vi "Take single measurement.vi"() -> ()   [LabVIEW 2017, in "GP22_TDC_Arduinoed.lvlib"]
uses:
  GP22_TDC_Arduinoed.lvlib
panel:
  out "error out":errorcluster
  out "Calibration / s":dbl format="%^#_6g"
  out "output / s":dbl format="%^#_6g"
  out "Self-Test Result Message":string
  in  "VISA resource name":refnum<visa-resource-name>
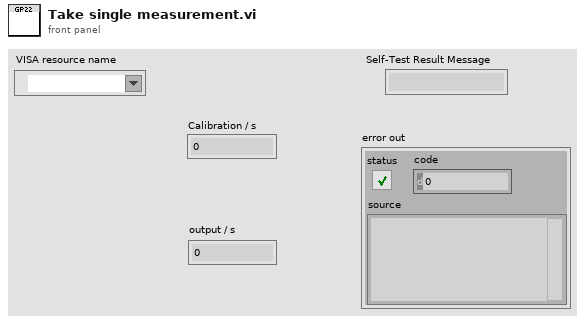
[diagram p1: front panel]
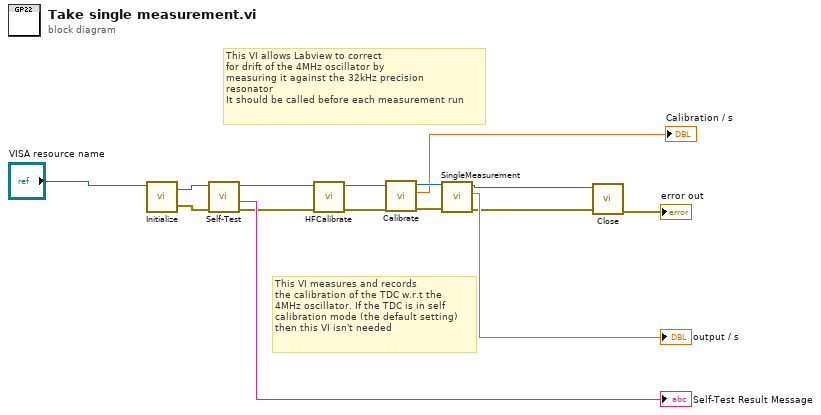
[diagram p0: block diagram]
diagram:
  # "This VI measures and records\nthe calibration of the TDC w.r.t the \n4MHz oscillator. If the TDC is in self \ncalibration mode (the default setting) \nthen this VI isn't needed"
  # "This VI allows Labview to correct\nfor drift of the 4MHz oscillator by\nmeasuring it against the 32kHz precision\nresonator\nIt should be called before each measurement run"
  n1 = call "Initialize.vi"("VISA resource name"="VISA resource name") -> ("error out"=w13:errorcluster, "VISA resource name out"=w14:refnum<visa-resource-name>)  [unwired: 5 in]
  n2 = call "Self-Test.vi"("error in (no error)"=w13, "VISA resource name"=w14) -> ("error out"=w3:errorcluster, "Self-Test Result Message"=→"Self-Test Result Message":string, "VISA resource name out"=w2:refnum<visa-resource-name>)  [unwired: 6 in, 1 out]
  n3 = call "HFCalibrate.vi"("error in (no error)"=w3, "VISA resource name"=w2) -> ("error out"=w4:errorcluster, "VISA resource name out"=w5:refnum<visa-resource-name>)  [unwired: 5 in, 2 out]
  n4 = call "Calibrate.vi"("error in (no error)"=w4, "VISA resource name"=w5) -> ("error out"=w8:errorcluster, "output / s"=→"Calibration / s":dbl, "VISA resource name out"=w9:refnum<visa-resource-name>)  [unwired: 5 in, 1 out]
  n5 = call "SingleMeasurement.vi"("error in (no error)"=w8, "VISA resource name"=w9) -> ("error out"=w7:errorcluster, "output / s"=→"output / s":dbl, "VISA resource name out"=w11:refnum<visa-resource-name>)  [unwired: 7 in]
  n6 = call "Close.vi"("error in (no error)"=w7, "VISA resource name"=w11) -> ("error out"=→"error out":errorcluster)  [unwired: 9 in]
